vi "update graph indicator.vi"(8 "customViData in":T1, 10 "plot":cluster{"X":u16[], "Y":u16[], "Y2":u16[]}) -> (0 "customViData out":T1)   [LabVIEW 2018]
uses:
  customViData.ctl
panel:
  out "plots":string[](array[string])
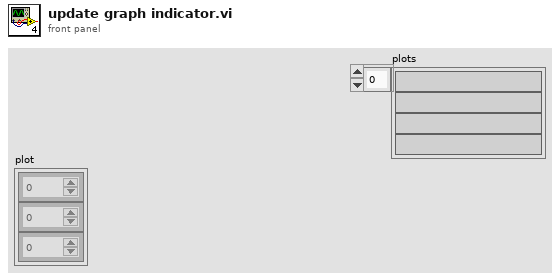
[diagram p1: front panel]
types:
  T1 = typedef "customViData.ctl" = cluster{"rigChannels":string[], "rigUnits":string[], "logging":bool, "plot":cluster{"X":u16[], "Y":u16[], "Y2":u16[]}, "updatePlot":bool, "chartRef":refnum<vi>, "livePlot":bool, "history":dbl[][], "channelCount":i32, "trendIndex":i32}
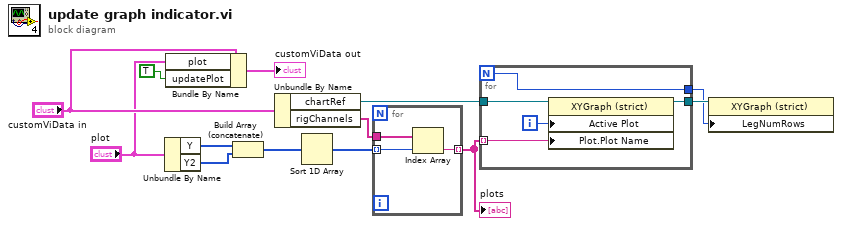
[diagram p0: block diagram]
diagram:
  n1 = Unbundle By Name("plot") -> ("Y"=w6:u16[], "Y2"=w5:u16[])
  n2 = Bundle By Name(cluster="customViData in", "plot"="plot", "updatePlot"=TRUE) -> (→"customViData out":T1)
  n3 = Build Array (concatenate)(w6, w5) -> (w4:u16[])
  n4 = Unbundle By Name("customViData in") -> ("chartRef"=w2:refnum<vi>, "rigChannels"=w10:string[])
  n5 = Sort 1D Array(array=w4) -> (sorted array=w3:u16[])
  n6 = for {
    tunnel: w10 -> [w16]
    tunnel: w3 -> [w15] mode=indexing
    tunnel: [w14] -> w9 mode=indexing
    n7 = Index Array(array=w16, index=w15) -> (element=w14:string)
  }
  "plots" <- w9
  n8 = for {
    N -> [w17]
    tunnel: w2 -> [w21]
    tunnel: w9 -> [w19] mode=indexing
    tunnel: [w18] -> w8
    tunnel: [w17] -> w7
    i -> [w20]
    n9 = property class="XYGraph (strict)"(reference=w21, "Active Plot"=w20, "Plot.Plot Name"=w19) -> (reference out=w18:refnum<vi>)  [unwired: 1 in, 1 out]
  }
  n10 = property class="XYGraph (strict)"(reference=w8, "LegNumRows"=w7) -> ()  [unwired: 1 in, 2 out]
